vi "FrontSight.vi"(1 "IMAQImage":T1) -> (0 "Image Out":T1)   [LabVIEW 2016, in "CCD monitor.lvlib" / "CCD monitor.lvclass"]
uses:
  <userlib>/Common Components/Hardware/Abstract System/Monitor/CCD monitor.lvclass
  <vilib>/vision/Image Controls.llb/IMAQ Image.ctl
  <resource>/objmgr/IMAQImage.rc
  <vilib>/vision/NI_Vision_Development_Module.lvlib
panel:
  out "Image":T1(plugin-control)
  in  "Bounding Rectangle":T2
  out "Image Size":cluster{"x":i32, "y":i32}
  in  "End Point 2":cluster{"X":i32, "Y":i32}
  in  "Color":u32(colorbox)=16711680
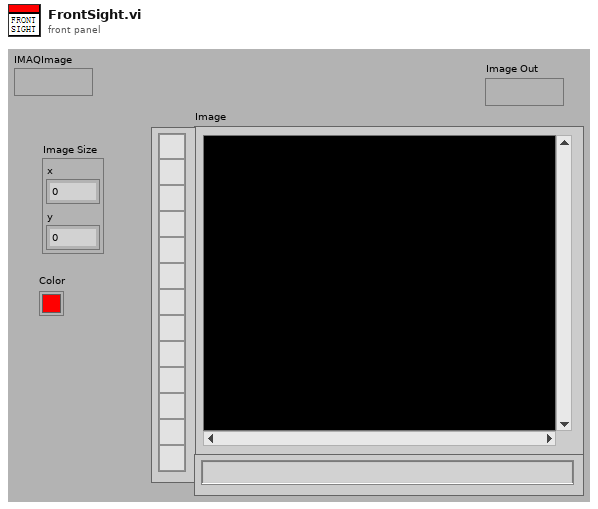
[diagram p1: front panel]
types:
  T1 = typedef "IMAQ Image.ctl" = refnum<image>
  T2 = cluster{"Left":i32, "Top":i32, "Right":i32, "Bottom":i32}
  T3 = cluster{"Desired Font (Application)":enum16{"User-specified Font", "Application Font", "System Font", "Dialog Font"}, "[User-specified Font]":cluster{"Font Name":string, "Size":i16, "Strikeout?":bool, "Italic?":bool, "Underline?":bool, "Outline?":bool, "Shadow?":bool, "Bold?":bool, "Rotation Angle":dbl}, "Horizontal Alignment":i16, "Vertical Alignment":i16}
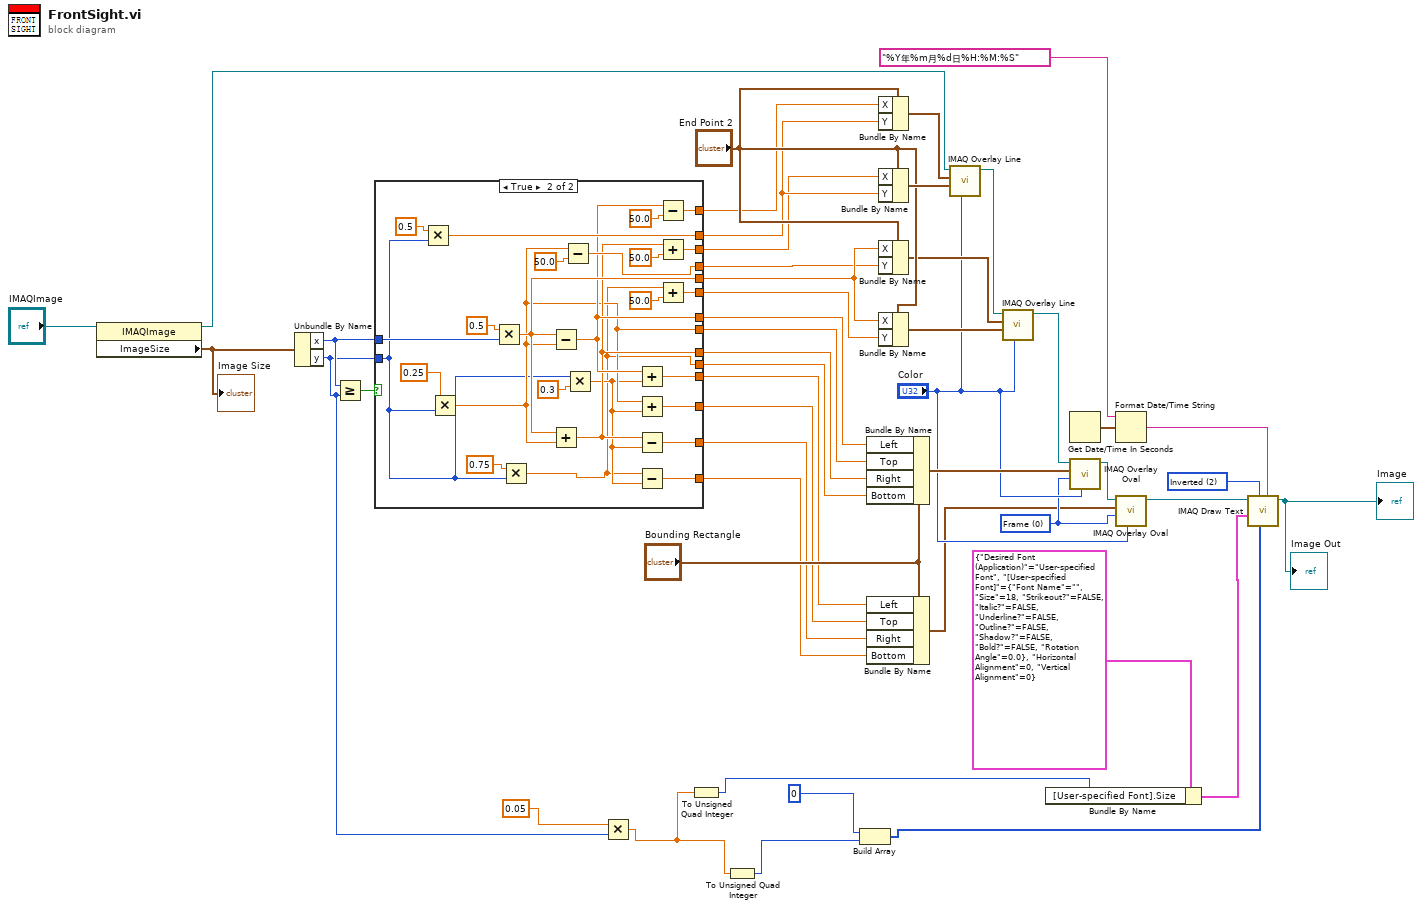
[diagram p0: block diagram]
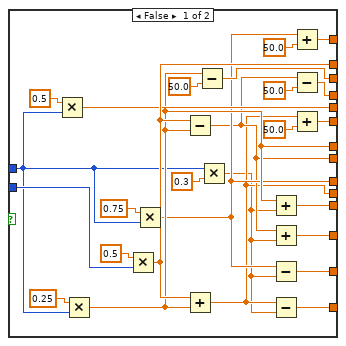
[diagram p2: hidden frame]
diagram:
  w12 = 2 items=["White", "Black", "Inverted", "Black on White", "White on Black"] ("Color")
  w27 = u32 0 items=["Frame", "Fill"] ("Drawing Mode (Frame)")
  n1 = property class="IMAQImage"(reference="IMAQImage") -> (reference out=w30:T1, "ImageSize"=w45:cluster{"x":i32, "y":i32})  [unwired: 1 in, 1 out]
  "Image Size" <- w45
  n2 = Unbundle By Name(w45) -> ("x"=w43:i32, "y"=w7:i32)
  n3 = Greater Or Equal?(x=w43, y=w7) -> (x >= y?=w42:bool)
  n4 = case shown="True" w42 {
    tunnel: w43 -> [w51 w98]
    tunnel: w7 -> [w71 w78]
    tunnel: [w54 w79] -> w37
    tunnel: [w60 w85] -> w41
    tunnel: [w55 w83] -> w31
    tunnel: [w53 w75] -> w36
    tunnel: [w70 w86] -> w33
    tunnel: [w69 w95] -> w32
    tunnel: [w63 w92] -> w26
    tunnel: [w64 w91] -> w25
    tunnel: [w62 w88] -> w24
    tunnel: [w61 w87] -> w23
    tunnel: [w59 w84] -> w20
    tunnel: [w58 w82] -> w19
    tunnel: [w57 w81] -> w18
    tunnel: [w56 w80] -> w17
    frame False {
      n5 = Multiply(x=0.5, y=w51) -> (x*y=w69:dbl)
      n6 = Multiply(x=0.25, y=w51) -> (x*y=w60:dbl)
      n7 = Multiply(x=0.5, y=w71) -> (x*y=w70:dbl)
      n8 = Multiply(x=0.75, y=w51) -> (x*y=w55:dbl)
      n9 = Subtract(x=w70, y=w60) -> (x-y=w54:dbl)
      n10 = Add(x=w70, y=w60) -> (x+y=w53:dbl)
      n11 = Subtract(x=w60, y=50.0) -> (x-y=w64:dbl)
      n12 = Multiply(x=w51, y=0.3) -> (x*y=w50:dbl)
      n13 = Add(x=w60, y=w50) -> (x+y=w59:dbl)
      n14 = Add(x=w54, y=w50) -> (x+y=w57:dbl)
      n15 = Subtract(x=w55, y=w50) -> (x-y=w58:dbl)
      n16 = Subtract(x=w53, y=w50) -> (x-y=w56:dbl)
      n17 = Add(x=w55, y=50.0) -> (x+y=w63:dbl)
      n18 = Subtract(x=w54, y=50.0) -> (x-y=w62:dbl)
      n19 = Add(x=w53, y=50.0) -> (x+y=w61:dbl)
    }
    frame True {
      n20 = Multiply(x=0.5, y=w78) -> (x*y=w86:dbl)
      n21 = Multiply(x=0.25, y=w78) -> (x*y=w79:dbl)
      n22 = Multiply(x=0.5, y=w98) -> (x*y=w95:dbl)
      n23 = Multiply(x=0.75, y=w78) -> (x*y=w75:dbl)
      n24 = Subtract(x=w95, y=w79) -> (x-y=w85:dbl)
      n25 = Add(x=w95, y=w79) -> (x+y=w83:dbl)
      n26 = Subtract(x=w79, y=50.0) -> (x-y=w88:dbl)
      n27 = Multiply(x=w78, y=0.3) -> (x*y=w77:dbl)
      n28 = Add(x=w85, y=w77) -> (x+y=w84:dbl)
      n29 = Add(x=w79, y=w77) -> (x+y=w81:dbl)
      n30 = Subtract(x=w83, y=w77) -> (x-y=w82:dbl)
      n31 = Subtract(x=w75, y=w77) -> (x-y=w80:dbl)
      n32 = Subtract(x=w85, y=50.0) -> (x-y=w92:dbl)
      n33 = Add(x=w83, y=50.0) -> (x+y=w91:dbl)
      n34 = Add(x=w75, y=50.0) -> (x+y=w87:dbl)
    }
  }
  n35 = Multiply(x=0.05, y=w7) -> (x*y=w2:dbl)
  n36 = To Unsigned Quad Integer(1:w2) -> (0:w1:u64)
  n37 = To Unsigned Quad Integer(1:w2) -> (0:w3:u64)
  n38 = Build Array(0, w3) -> (w8:u64[])
  n39 = Bundle By Name(cluster="Bounding Rectangle", "Left"=w41, "Top"=w37, "Right"=w31, "Bottom"=w36) -> (w44:T2)
  n40 = Bundle By Name(cluster="Bounding Rectangle", "Left"=w20, "Top"=w18, "Right"=w19, "Bottom"=w17) -> (w21:T2)
  n41 = Bundle By Name(cluster="End Point 2", "X"=w26, "Y"=w33) -> (w40:cluster{"X":i32, "Y":i32})
  n42 = Bundle By Name(cluster="End Point 2", "X"=w25, "Y"=w33) -> (w39:cluster{"X":i32, "Y":i32})
  n43 = Bundle By Name(cluster="End Point 2", "X"=w32, "Y"=w24) -> (w35:cluster{"X":i32, "Y":i32})
  n44 = Bundle By Name(cluster="End Point 2", "X"=w32, "Y"=w23) -> (w34:cluster{"X":i32, "Y":i32})
  n45 = call "IMAQ Overlay Line"("Color"="Color", "End Point"=w39, "Start Point"=w40, "Image"=w30) -> ("Image Out"=w47:T1)  [unwired: 6 in, 1 out]
  n46 = call "IMAQ Overlay Line"("Color"="Color", "End Point"=w34, "Start Point"=w35, "Image"=w47) -> ("Image Out"=w46:T1)  [unwired: 6 in, 1 out]
  n47 = Bundle By Name(cluster=T3 {"Desired Font (Application)"=enum."User-specified Font", "[User-specified Font]"={"Font Name"="", "Size"=18, "Strikeout?"=FALSE, "Italic?"=FALSE, "Underline?"=FALSE, "Outline?"=FALSE, "Shadow?"=FALSE, "Bold?"=FALSE, "Rotation Angle"=0.0}, "Horizontal Alignment"=0, "Vertical Alignment"=0} ("Font, Size & Style"), "[User-specified Font].Size"=w1) -> (w5:T3)
  n48 = Get Date/Time In Seconds() -> (seconds since 1Jan1904=w15:timestamp)
  n49 = call "IMAQ Overlay Oval"("Color"="Color", "Drawing Mode (Frame)"=w27, "Bounding Rectangle"=w44, "Image"=w46) -> ("Image Out"=w29:T1)  [unwired: 6 in, 1 out]
  n50 = Format Date/Time String(time format string (%c)="%Y年%m月%d日%H:%M:%S" ("时间格式字符串(%c)"), seconds (now)=w15) -> (date/time string=w13:string)  [unwired: 1 in]
  n51 = call "IMAQ Overlay Oval"("Color"="Color", "Drawing Mode (Frame)"=w27, "Bounding Rectangle"=w21, "Image"=w29) -> ("Image Out"=w11:T1)  [unwired: 6 in, 1 out]
  n52 = call "IMAQ Draw Text"("String"=w13, "Insertion Point"=w8, "Color"=w12, "Font, Size & Style"=w5, "Image Src"=w11) -> ("Image Dst Out"=→"Image" →"Image Out":T1)  [unwired: 3 in, 3 out]
